vi "mono_send_simulator_config.vi"(4 "error in":errorcluster, 6 "Simulator Configuration Path":path, 7 "monoDrive Connection In":refnum<k5>) -> (0 "error out":errorcluster, 1 "monoDrive Connection Out":refnum<k5>, 3 "response":string)   [LabVIEW 2018, in "monoDrive.lvlib"]
uses:
  monoDrive.lvlib
  Simulator_Configuration.ctl
  mono_commands.ctl
panel:
  in  "enable LabVIEW extensions? (T)":bool
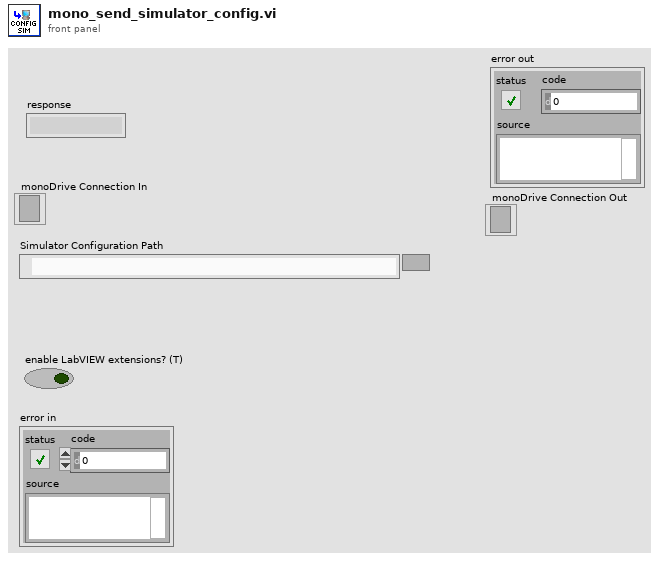
[diagram p1: front panel]
types:
  T1 = typedef "monoDrive.lvlib/mono_commands.ctl" = cluster{"SIMULATOR_STATUS_UUID":string, "STREAM_DATA_COMMAND_UUID":string, "SIMULATOR_CONFIG_COMMAND_UUID":string, "VEHICLE_CONFIG_COMMAND_UUID":string, "EGO_CONTROL_COMMAND_UID":string, "WAYPOINT_UPDATE_COMMAND_UID":string, "SCENARIO_COMMAND_UID":string, "MAP_COMMAND_UID":string, "SPAWN_COMMAND_UID":string, "MOVE_ACTOR_COMMAND_UID":string, "SCENARIO_INIT_COMMAND_UID":string, "ATTACH_SENSOR_COMMAND_UID":string, "DETACH_SENSOR_COMMAND_UID":string, "CONTROL_HEADER":string, "RESPONSE_HEADER":string}
  T2 = typedef "Simulator_Configuration.ctl" = cluster{"id":string, "server_ip":string, "server_port":i32, "client_ip":string, "phys_materials":cluster{"Aluminum":cluster{"specular_exponent":i32, "specular_coefficient":i32, "diffuse_coefficient":i32, "dielectric_constant":i32, "roughness":i32}, "Asphalt":cluster{"specular_exponent":i32, "specular_coefficient":i32, "diffuse_coefficient":i32, "dielectric_constant":i32, "roughness":i32}, "Road":cluster{"specular_exponent":i32, "specular_coefficient":i32, "diffuse_coefficient":i32, "dielectric_constant":i32, "roughness":i32}, "Concrete":cluster{"specular_exponent":i32, "specular_coefficient":i32, "diffuse_coefficient":i32, "dielectric_constant":i32, "roughness":i32}, "Glass":cluster{"specular_exponent":i32, "specular_coefficient":i32, "diffuse_coefficient":i32, "dielectric_constant":i32, "roughness":i32}, "LandScape":cluster{"specular_exponent":i32, "specular_coefficient":i32, "diffuse_coefficient":i32, "dielectric_constant":i32, "roughness":i32}, "Plastic":cluster{"specular_exponent":i32, "specular_coefficient":i32, "diffuse_coefficient":i32, "dielectric_constant":i32, "roughness":i32}, "Steel":cluster{"specular_exponent":i32, "specular_coefficient":i32, "diffuse_coefficient":i32, "dielectric_constant":i32, "roughness":i32}, "Tree":cluster{"specular_exponent":i32, "specular_coefficient":i32, "diffuse_coefficient":i32, "dielectric_constant":i32, "roughness":i32}, "Wheel":cluster{"specular_exponent":i32, "specular_coefficient":i32, "diffuse_coefficient":i32, "dielectric_constant":i32, "roughness":i32}, "Tire":cluster{"specular_exponent":i32, "specular_coefficient":i32, "diffuse_coefficient":i32, "dielectric_constant":i32, "roughness":i32}}, "traffic_configuration":cluster{"max_vehicles":i32, "spawn_rate":i32}, "client_settings":cluster{"map":cluster{"gis_anchor":cluster{"x":i32, "y":i32, "z":i32}, "point_delta":i32}, "gui":cluster{"fps":i32}, "logger":cluster{"sensor":string, "network":string, "control":string, "scenario":string, "simulator":string, "vehicle":string}}}
  T3 = cluster{"type":string, "success":bool, "message":T2}
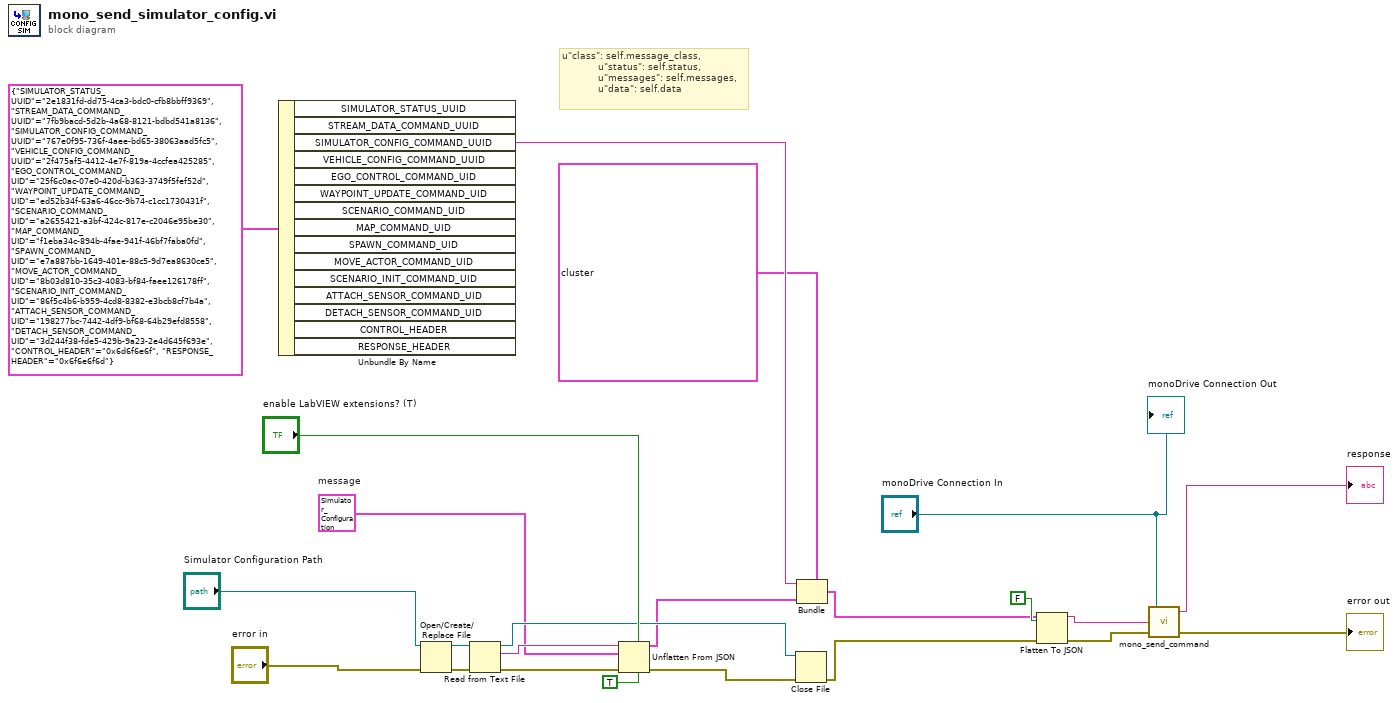
[diagram p0: block diagram]
diagram:
  w14 = T2 {"id"="", "server_ip"="", "server_port"=0, "client_ip"="", "phys_materials"={"Aluminum"={"specular_exponent"=0, "specular_coefficient"=0, "diffuse_coefficient"=0, "dielectric_constant"=0, "roughness"=0}, "Asphalt"={"specular_exponent"=0, "specular_coefficient"=0, "diffuse_coefficient"=0, "dielectric_constant"=0, "roughness"=0}, "Road"={"specular_exponent"=0, "specular_coefficient"=0, "diffuse_coefficient"=0, "dielectric_constant"=0, "roughness"=0}, "Concrete"={"specular_exponent"=0, "specular_coefficient"=0, "diffuse_coefficient"=0, "dielectric_constant"=0, "roughness"=0}, "Glass"={"specular_exponent"=0, "specular_coefficient"=0, "diffuse_coefficient"=0, "dielectric_constant"=0, "roughness"=0}, "LandScape"={"specular_exponent"=0, "specular_coefficient"=0, "diffuse_coefficient"=0, "dielectric_constant"=0, "roughness"=0}, "Plastic"={"specular_exponent"=0, "specular_coefficient"=0, "diffuse_coefficient"=0, "dielectric_constant"=0, "roughness"=0}, "Steel"={"specular_exponent"=0, "specular_coefficient"=0, "diffuse_coefficient"=0, "dielectric_constant"=0, "roughness"=0}, "Tree"={"specular_exponent"=0, "specular_coefficient"=0, "diffuse_coefficient"=0, "dielectric_constant"=0, "roughness"=0}, "Wheel"={"specular_exponent"=0, "specular_coefficient"=0, "diffuse_coefficient"=0, "dielectric_constant"=0, "roughness"=0}, "Tire"={"specular_exponent"=0, "specular_coefficient"=0, "diffuse_coefficient"=0, "dielectric_constant"=0, "roughness"=0}}, "traffic_configuration"={"max_vehicles"=0, "spawn_rate"=0}, "client_settings"={"map"={"gis_anchor"={"x"=0, "y"=0, "z"=0}, "point_delta"=0}, "gui"={"fps"=0}, "logger"={"sensor"="", "network"="", "control"="", "scenario"="", "simulator"="", "vehicle"=""}}}  # message
  # "u\"class\": self.message_class,\n            u\"status\": self.status,\n            u\"messages\": self.messages,\n            u\"data\": self.data"
  n1 = Unbundle By Name(T1 {"SIMULATOR_STATUS_UUID"="2e1831fd-dd75-4ca3-bdc0-cfb8bbff9369", "STREAM_DATA_COMMAND_UUID"="7fb9bacd-5d2b-4a68-8121-bdbd541a8136", "SIMULATOR_CONFIG_COMMAND_UUID"="767e0f95-736f-4aee-bd65-38063aad5fc5", "VEHICLE_CONFIG_COMMAND_UUID"="2f475af5-4412-4e7f-819a-4ccfea425285", "EGO_CONTROL_COMMAND_UID"="25f6c0ac-07e0-420d-b363-3749f5fef52d", "WAYPOINT_UPDATE_COMMAND_UID"="ed52b34f-63a6-46cc-9b74-c1cc1730431f", "SCENARIO_COMMAND_UID"="a2655421-a3bf-424c-817e-c2046e95be30", "MAP_COMMAND_UID"="f1eba34c-894b-4fae-941f-46bf7faba0fd", "SPAWN_COMMAND_UID"="e7a887bb-1649-401e-88c5-9d7ea8630ce5", "MOVE_ACTOR_COMMAND_UID"="8b03d810-35c3-4083-bf84-faee126178ff", "SCENARIO_INIT_COMMAND_UID"="86f5c4b6-b959-4cd8-8382-e3bcb8cf7b4a", "ATTACH_SENSOR_COMMAND_UID"="198277bc-7442-4df9-bf68-64b29efd8558", "DETACH_SENSOR_COMMAND_UID"="3d244f38-fde5-429b-9a23-2e4d645f693e", "CONTROL_HEADER"="0x6d6f6e6f", "RESPONSE_HEADER"="0x6f6e6f6d"} ("Cluster")) -> ("SIMULATOR_CONFIG_COMMAND_UUID"=w11:string)  [unwired: 14 out]
  n2 = Open/Create/Replace File(file path (use dialog)="Simulator Configuration Path", error in="error in") -> (refnum out=w16:refnum<file>, error out=w17:errorcluster)  [unwired: 4 in, 1 out]
  n3 = Read from Text File(file (use dialog)=w16, error in=w17) -> (refnum out=w20:refnum<file>, text=w22:string, error out=w19:errorcluster)  [unwired: 2 in, 1 out]
  n4 = Unflatten From JSON(enable LabVIEW extensions? (T)="enable LabVIEW extensions? (T)", JSON string=w22, type and defaults=w14, strict validation? (F)=TRUE, error in (no error)=w19) -> (value=w2:T2, error out=w18:errorcluster)  [unwired: 2 in]
  n5 = Close File(refnum=w20, error in=w18) -> (error out=w6:errorcluster)  [unwired: 1 out]
  n6 = Bundle(cluster=T3 {"type"="", "success"=TRUE, "message"={"id"="", "server_ip"="", "server_port"=0, "client_ip"="", "phys_materials"={"Aluminum"={"specular_exponent"=0, "specular_coefficient"=0, "diffuse_coefficient"=0, "dielectric_constant"=0, "roughness"=0}, "Asphalt"={"specular_exponent"=0, "specular_coefficient"=0, "diffuse_coefficient"=0, "dielectric_constant"=0, "roughness"=0}, "Road"={"specular_exponent"=0, "specular_coefficient"=0, "diffuse_coefficient"=0, "dielectric_constant"=0, "roughness"=0}, "Concrete"={"specular_exponent"=0, "specular_coefficient"=0, "diffuse_coefficient"=0, "dielectric_constant"=0, "roughness"=0}, "Glass"={"specular_exponent"=0, "specular_coefficient"=0, "diffuse_coefficient"=0, "dielectric_constant"=0, "roughness"=0}, "LandScape"={"specular_exponent"=0, "specular_coefficient"=0, "diffuse_coefficient"=0, "dielectric_constant"=0, "roughness"=0}, "Plastic"={"specular_exponent"=0, "specular_coefficient"=0, "diffuse_coefficient"=0, "dielectric_constant"=0, "roughness"=0}, "Steel"={"specular_exponent"=0, "specular_coefficient"=0, "diffuse_coefficient"=0, "dielectric_constant"=0, "roughness"=0}, "Tree"={"specular_exponent"=0, "specular_coefficient"=0, "diffuse_coefficient"=0, "dielectric_constant"=0, "roughness"=0}, "Wheel"={"specular_exponent"=0, "specular_coefficient"=0, "diffuse_coefficient"=0, "dielectric_constant"=0, "roughness"=0}, "Tire"={"specular_exponent"=0, "specular_coefficient"=0, "diffuse_coefficient"=0, "dielectric_constant"=0, "roughness"=0}}, "traffic_configuration"={"max_vehicles"=0, "spawn_rate"=0}, "client_settings"={"map"={"gis_anchor"={"x"=0, "y"=0, "z"=0}, "point_delta"=0}, "gui"={"fps"=0}, "logger"={"sensor"="", "network"="", "control"="", "scenario"="", "simulator"="", "vehicle"=""}}}}, "type"=w11, "message"=w2) -> (w3:T3)  [unwired: 1 in]
  n7 = Flatten To JSON(enable LabVIEW extensions? (T)=FALSE, anything=w3, error in (no error)=w6) -> (JSON string=w8:string, 11:w7:errorcluster)
  n8 = call "mono_send_command.vi"("error in (no error)"=w7, "JSON Command"=w8, "TCP Network Connection in"="monoDrive Connection In") -> ("error out"=→"error out":errorcluster, "response"=→"response":string)  [unwired: 1 in]
  "monoDrive Connection Out" <- "monoDrive Connection In"
